vi "Configure Clock (5761).vi"(7 "Timeout (s)":dbl=5.0 caption="Time Target (s)", 8 "error in":errorcluster, 10 "Sample Clock Select":u8=3, 11 "FPGA Session":T1) -> (0 "error out":errorcluster, 2 "Configuration Error":bool, 3 "FPGA Session":T1, 4 "timedout?":bool, 6 "io mod.synthesizer locked":bool)   [LabVIEW 2011, in "FlexRIO Host Library (User).lvlib"]
doc: "This VI is used to configure the clock\n\n0 -- Oscillator on 5761\n1 -- \n2 --\n3 -- Oscillator on 5761 locked to Back plane 10MHz"
uses:
  FlexRIO Host Library (User).lvlib
  <vilib>/rvi/interface/nirviReadWriteControl/nirviReadWriteControl.xnode
  Session/FPGA Session Ref.ctl
  OCT Reference Design/FPGA Bitfiles/OCTDigitizer_FPGABoard_AcquireDatawitho_CC2D8059.lvbitx
  OCT Reference Design/Complete FPGA Engine/Acquire Data without DRAM.vi
  <vilib>/rvi/errors/niLvFpgaAdjustHostInterfaceError.vi
panel:
  out "Elapsed Time (s)":dbl
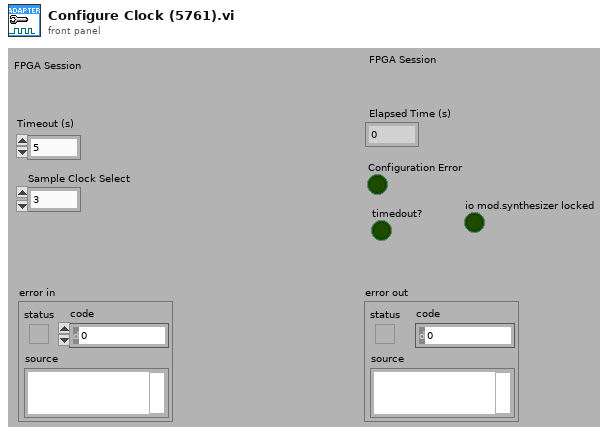
[diagram p1: front panel]
types:
  T1 = typedef "FlexRIO Host Library (User).lvlib/FPGA Session Ref.ctl" = refnum<k20>
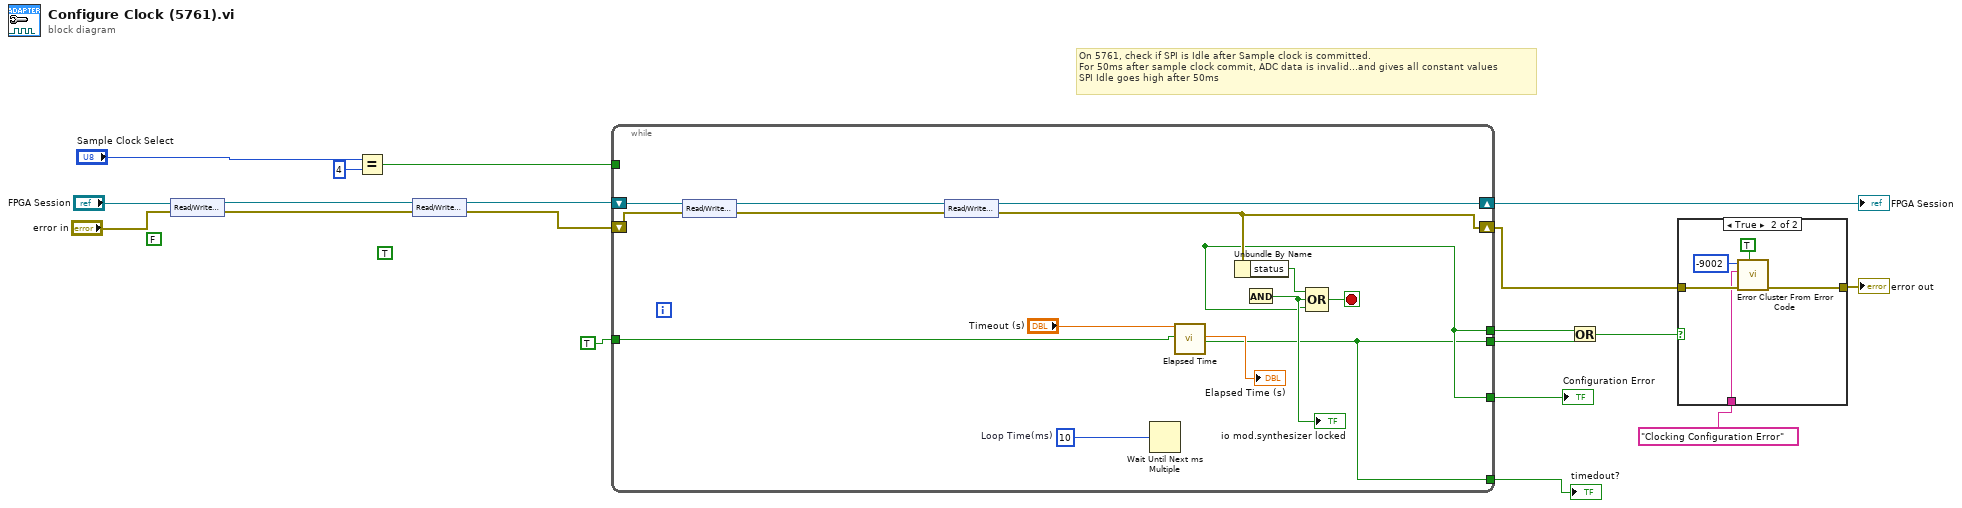
[diagram p0: block diagram]
diagram:
  w6 = FALSE ("io mod.sample clock commit")
  w7 = TRUE ("io mod.sample clock commit")
  # "On 5761, check if SPI is Idle after Sample clock is committed.\nFor 50ms after sample clock commit, ADC data is invalid...and gives all constant values\nSPI Idle goes high after 50ms"
  n1 = xnode "Read/Write Control"("FPGA VI Reference In"="FPGA Session", "error in"="error in") -> ("FPGA VI Reference Out"=w13:T1, "error out"=w12:errorcluster)
  n2 = Equal?(x="Sample Clock Select", y=u8 4) -> (x = y?=w3:bool)
  n3 = xnode "Read/Write Control"("FPGA VI Reference In"=w13, "error in"=w12) -> ("FPGA VI Reference Out"=w11:T1, "error out"=w10:errorcluster)
  n4 = while {
    shift-right: [w32] -> w21
    shift-left: w10 -> [w29]
    tunnel: [w22] -> w17
    shift-right: [w33] -> w15
    shift-left: w11 -> [w30]
    tunnel: TRUE ("Reset") -> [w31]
    tunnel: [w23] -> w8
    tunnel: w3 -> [_]
    tunnel: [w23] -> w2
    tunnel: [w22] -> w1
    stop <- w37 stop-if-true
    w38 = u32 10  # Loop Time(ms)
    n5 = xnode "Read/Write Control"("FPGA VI Reference In"=w30, "error in"=w29) -> ("FPGA VI Reference Out"=w28:T1, "error out"=w27:errorcluster)
    n6 = xnode "Read/Write Control"("FPGA VI Reference In"=w28, "error in"=w27) -> ("FPGA VI Reference Out"=w33:T1, "error out"=w32:errorcluster)
    n7 = Wait Until Next ms Multiple(millisecond multiple=w38) -> ()  [unwired: 1 out]
    n8 = call "Elapsed Time"("Time Target (s)"="Timeout (s)", "Reset"=w31) -> ("Elapsed Time (s)"=→"Elapsed Time (s)":dbl, "Time has Elapsed"=w22:bool)  [unwired: 10 in, 6 out]
    n9 = Unbundle By Name(w32) -> ("status"=w36:bool)
    n10 = And() -> (x=w26:bool, y=w25:bool, x .and. y?=w24:bool)
    "io mod.synthesizer locked" <- w24
    n11 = Compound Arithmetic op=OR(w36, w24) -> (w37:bool, w23:bool)
  }
  "FPGA Session" <- w15
  "Configuration Error" <- w2
  "timedout?" <- w1
  n12 = Or(x=w8, y=w17) -> (x .or. y?=w16:bool)
  n13 = case shown="True" w16 {
    tunnel: w21 -> [w39 w43]
    tunnel: [w39 w42] -> w14
    tunnel: "Clocking Configuration Error" ("Error Message") -> [_ w41]
    frame False {
    }
    frame True {
      n14 = call <vilib>:"Error Cluster From Error Code.vi"("show call chain? (False)"=TRUE, "error in (no error)"=w43, "error message (\"\")"=w41, "error code (0)"=-9002) -> ("error out"=w42:errorcluster)  [unwired: 5 in]
    }
  }
  "error out" <- w14
